vi "tdms.vi"   [LabVIEW 2016]
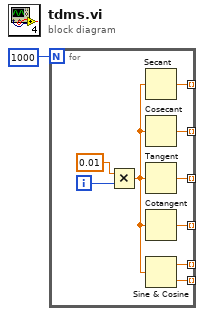
[diagram p0: block diagram]
diagram:
  n1 = for {
    N: 1000 -> [_]
    tunnel: [w7] -> _ mode=indexing
    tunnel: [w6] -> _ mode=indexing
    tunnel: [w5] -> _ mode=indexing
    tunnel: [w4] -> _ mode=indexing
    tunnel: [w3] -> _ mode=indexing
    tunnel: [w2] -> _ mode=indexing
    i -> [w10]
    n2 = Multiply(x=0.01, y=w10) -> (x*y=w8:dbl)
    n3 = Secant(1:w8) -> (0:w5:dbl)
    n4 = Cosecant(1:w8) -> (0:w4:dbl)
    n5 = Tangent(1:w8) -> (0:w3:dbl)
    n6 = Cotangent(1:w8) -> (0:w2:dbl)
    n7 = Sine & Cosine(0:w8) -> (1:w7:dbl, 2:w6:dbl)
  }
